vi "Adder4.vi"() -> (8 "Adder4":refnum<class "Adder4.lvclass">)   [LabVIEW 2017, in "Adder4.lvclass"]
uses:
  Adder4.lvclass
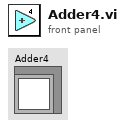
[diagram p1: front panel]
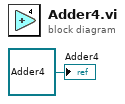
[diagram p0: block diagram]
diagram:
  "Adder4" <- refnum<class "Adder4.lvclass"> refnum ("Adder4.lvclass")
